vi "Year2017_Question3.vi"() -> ()   [LabVIEW 2015]
panel:
  out "Average":dbl
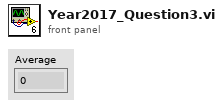
[diagram p1: front panel]
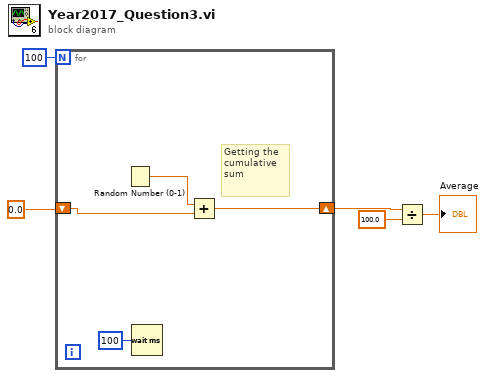
[diagram p0: block diagram]
diagram:
  n1 = for {
    N: 100 -> [_]
    shift-right: [w7] -> w1
    shift-left: 0.0 ("number: 0 to 1") -> [w6]
    # "Getting the\ncumulative\nsum"
    n2 = Random Number (0-1)() -> (number: 0 to 1=w9:dbl)
    n3 = Wait (ms)(milliseconds to wait=u32 100) -> ()  [unwired: 1 out]
    n4 = Add(x=w9, y=w6) -> (x+y=w7:dbl)
  }
  n5 = Divide(x=w1, y=100.0) -> (x/y=→"Average":dbl)
